vi "create_instrument_semaphores.vi"(11 "instrument array in":refnum<class "instrument.lvclass">[](array[class])) -> (3 "instrument array out":refnum<class "instrument.lvclass">[](array[class]))   [LabVIEW 2013]
doc: "input is array of instrument objects. Go through very object and create a semaphore for each object (the name of the semaphore is the name of the instrument object. out put is the same array of objects"
uses:
  Classes/Instrument/instrument.lvclass
panel:
  out "error out":errorcluster
  in  "error in (no error)":errorcluster
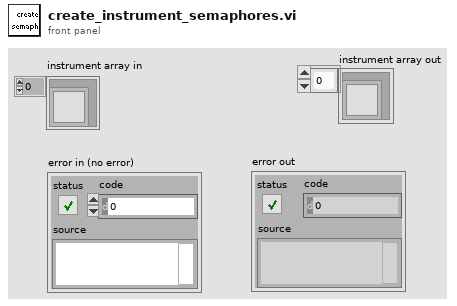
[diagram p1: front panel]
types:
  T1 = typedef "Semaphore RefNum" = refnum<k1>
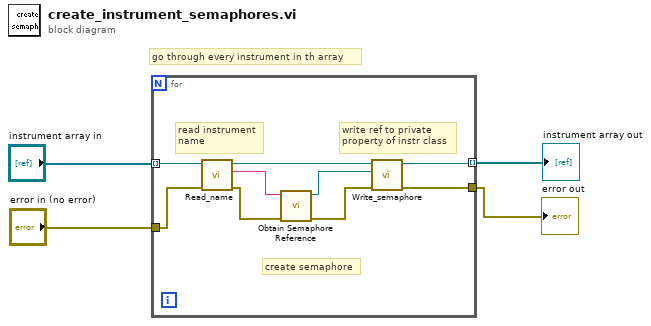
[diagram p0: block diagram]
diagram:
  # "go through every instrument in th array"
  n1 = for {
    tunnel: "instrument array in" -> [w13] mode=indexing
    tunnel: [w7] -> w2 mode=indexing
    tunnel: "error in (no error)" -> [w6]
    tunnel: [w5] -> w3
    # "write ref to private\nproperty of instr class"
    # "create semaphore"
    # "read instrument\nname"
    n2 = call-dynamic "Read_name.vi"("error in (no error)"=w6, "instrument in"=w13) -> ("error out"=w10:errorcluster, "name"=w11:string, "instrument out"=w12:refnum<class "instrument.lvclass">)  [unwired: 7 in]
    n3 = call <vilib>:"Obtain Semaphore Reference.vi"("error in (no error)"=w10, "name (unnamed)"=w11) -> ("error out"=w8:errorcluster, "semaphore"=w9:T1)  [unwired: 3 in, 1 out]
    n4 = call-dynamic "Write_semaphore.vi"("error in (no error)"=w8, "semaphore"=w9, "instrument in"=w12) -> ("error out"=w5:errorcluster, "instrument out"=w7:refnum<class "instrument.lvclass">)  [unwired: 7 in]
  }
  "error out" <- w3
  "instrument array out" <- w2
